vi "Write pOriginY.vi"(8 "error in (no error)":errorcluster, 10 "pOriginY":dbl[unit] min=-0.1 max=0.1, 11 "POrigin in":refnum<class "POrigin.lvclass">) -> (0 "error out":errorcluster, 3 "POrigin out":refnum<class "POrigin.lvclass">)   [LabVIEW 2014, in "TCSDataDefinitions.lvlib" / "TCSCommand.lvlib" / "POriginCommands.lvlib" / "POrigin.lvclass"]
uses:
  POrigin.lvclass
  POrigin.lvclass/POrigin.ctl
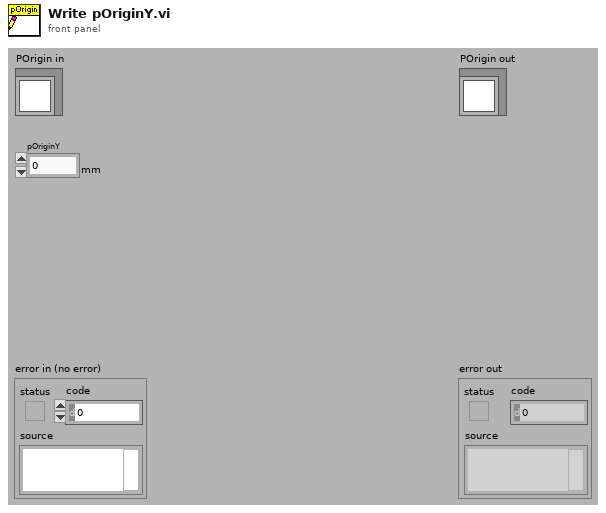
[diagram p1: front panel]
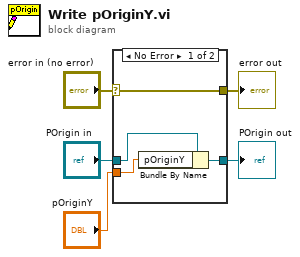
[diagram p0: block diagram]
diagram:
  n1 = case shown="No Error" "error in (no error)" {
    selector: "error in (no error)" -> [w9 w10]
    tunnel: [w9 w10] -> w4
    tunnel: [w7 w11] -> w2
    tunnel: "POrigin in" -> [w8 w11]
    tunnel: "pOriginY" -> [w6 _]
    frame No Error {
      n2 = Bundle By Name(cluster=w8, "pOriginY"=w6) -> (w7:refnum<class "POrigin.lvclass">)
    }
    frame Error {
    }
  }
  "error out" <- w4
  "POrigin out" <- w2
